vi "Test_Comunications.vi"() -> ()   [LabVIEW 2019]
panel:
  out "Vel_I":dbl
  out "Vel_D":dbl
  out "Distancia_ToF":dbl
  out "Ultrasonido_1":dbl
  out "Ultrasonido_2":dbl
  out "Trama Recibida":string
  in  "Servo_Gripper":dbl
  in  "Motor_Riel":dbl
  in  "Motor_I":dbl
  in  "Motor_D":dbl
  out "Trama de envío":string
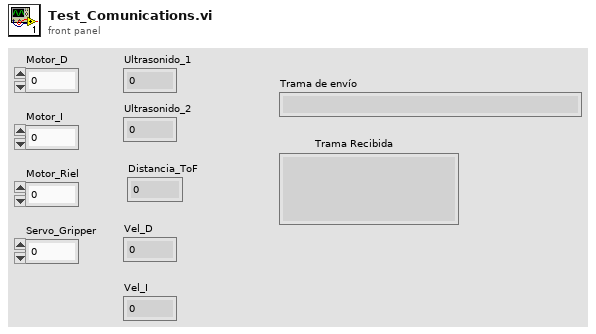
[diagram p1: front panel]
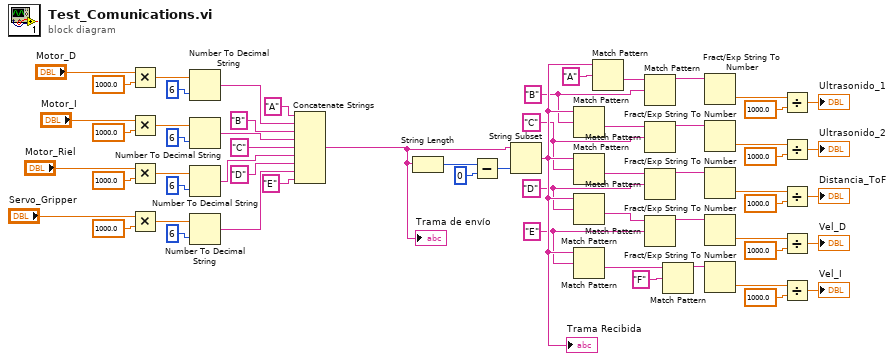
[diagram p0: block diagram]
diagram:
  w32 = "E" ("regular expression")
  w33 = "D" ("regular expression")
  w34 = "C" ("regular expression")
  w35 = "B" ("regular expression")
  n1 = Multiply(x="Motor_D", y=1000.0) -> (x*y=w30:dbl)
  n2 = Multiply(x="Motor_I", y=1000.0) -> (x*y=w24:dbl)
  n3 = Multiply(x="Motor_Riel", y=1000.0) -> (x*y=w23:dbl)
  n4 = Multiply(x="Servo_Gripper", y=1000.0) -> (x*y=w25:dbl)
  n5 = Number To Decimal String(number=w30, width (-)=i16 6) -> (decimal integer string=w53:string)
  n6 = Number To Decimal String(number=w24, width (-)=i16 6) -> (decimal integer string=w55:string)
  n7 = Number To Decimal String(number=w23, width (-)=i16 6) -> (decimal integer string=w57:string)
  n8 = Number To Decimal String(number=w25, width (-)=i16 6) -> (decimal integer string=w60:string)
  n9 = Concatenate Strings("A" ("string"), w53, "B" ("string"), w55, "C" ("string"), w57, "D" ("string"), w60, "E" ("string")) -> (w36:string)
  "Trama de envío" <- w36
  n10 = String Length(string=w36) -> (length=w38:i32)
  n11 = Subtract(x=w38, y=0) -> (x-y=w40:i32)
  n12 = String Subset(string=w36, length (rest)=w40) -> (substring=w37:string)  [unwired: 1 in]
  "Trama Recibida" <- w37
  n13 = Match Pattern(string=w37, regular expression=w35) -> (after substring=w48:string)  [unwired: 1 in, 3 out]
  n14 = Match Pattern(string=w37, regular expression=w34) -> (after substring=w47:string)  [unwired: 1 in, 3 out]
  n15 = Match Pattern(string=w37, regular expression=w33) -> (after substring=w44:string)  [unwired: 1 in, 3 out]
  n16 = Match Pattern(string=w37, regular expression=w32) -> (after substring=w43:string)  [unwired: 1 in, 3 out]
  n17 = Match Pattern(string=w37, regular expression="A") -> (after substring=w52:string)  [unwired: 1 in, 3 out]
  n18 = Match Pattern(string=w52, regular expression=w35) -> (before substring=w50:string)  [unwired: 1 in, 3 out]
  n19 = Match Pattern(string=w48, regular expression=w34) -> (before substring=w49:string)  [unwired: 1 in, 3 out]
  n20 = Match Pattern(string=w47, regular expression=w33) -> (before substring=w46:string)  [unwired: 1 in, 3 out]
  n21 = Match Pattern(string=w44, regular expression=w32) -> (before substring=w45:string)  [unwired: 1 in, 3 out]
  n22 = Match Pattern(string=w43, regular expression="F") -> (before substring=w41:string)  [unwired: 1 in, 3 out]
  n23 = Fract/Exp String To Number(string=w50) -> (number=w14:dbl)  [unwired: 3 in, 1 out]
  n24 = Fract/Exp String To Number(string=w49) -> (number=w8:dbl)  [unwired: 3 in, 1 out]
  n25 = Fract/Exp String To Number(string=w46) -> (number=w7:dbl)  [unwired: 3 in, 1 out]
  n26 = Fract/Exp String To Number(string=w45) -> (number=w6:dbl)  [unwired: 3 in, 1 out]
  n27 = Fract/Exp String To Number(string=w41) -> (number=w5:dbl)  [unwired: 3 in, 1 out]
  n28 = Divide(x=w14, y=1000.0) -> (x/y=→"Ultrasonido_1":dbl)
  n29 = Divide(x=w8, y=1000.0) -> (x/y=→"Ultrasonido_2":dbl)
  n30 = Divide(x=w7, y=1000.0) -> (x/y=→"Distancia_ToF":dbl)
  n31 = Divide(x=w6, y=1000.0) -> (x/y=→"Vel_D":dbl)
  n32 = Divide(x=w5, y=1000.0) -> (x/y=→"Vel_I":dbl)
